vi "Arm Motor Example.vi"() -> ()   [LabVIEW 2011]
panel:
  in  "Velocity":dbl(knob)=1.0440740470075023 scale=-10.0..10.0
  out "Motor Power":dbl(slide) scale=-1.0..1.0
  out "Waveform Chart":dbl(graph)
  in  "initialize":bool
  out "Position":dbl format="%0.2f"
  in  "Right/Up/CW Limit":dbl=10.0
  in  "Left/Dn/CCW Limit":dbl=-10.0
  in  "Joystick Input":dbl(slide)=0.005128205128205127 scale=-1.0..1.0
  out "Motor":dbl
  out "Read Right Limit":dbl=30.0
  out "Read Left Limit":dbl=-185.0
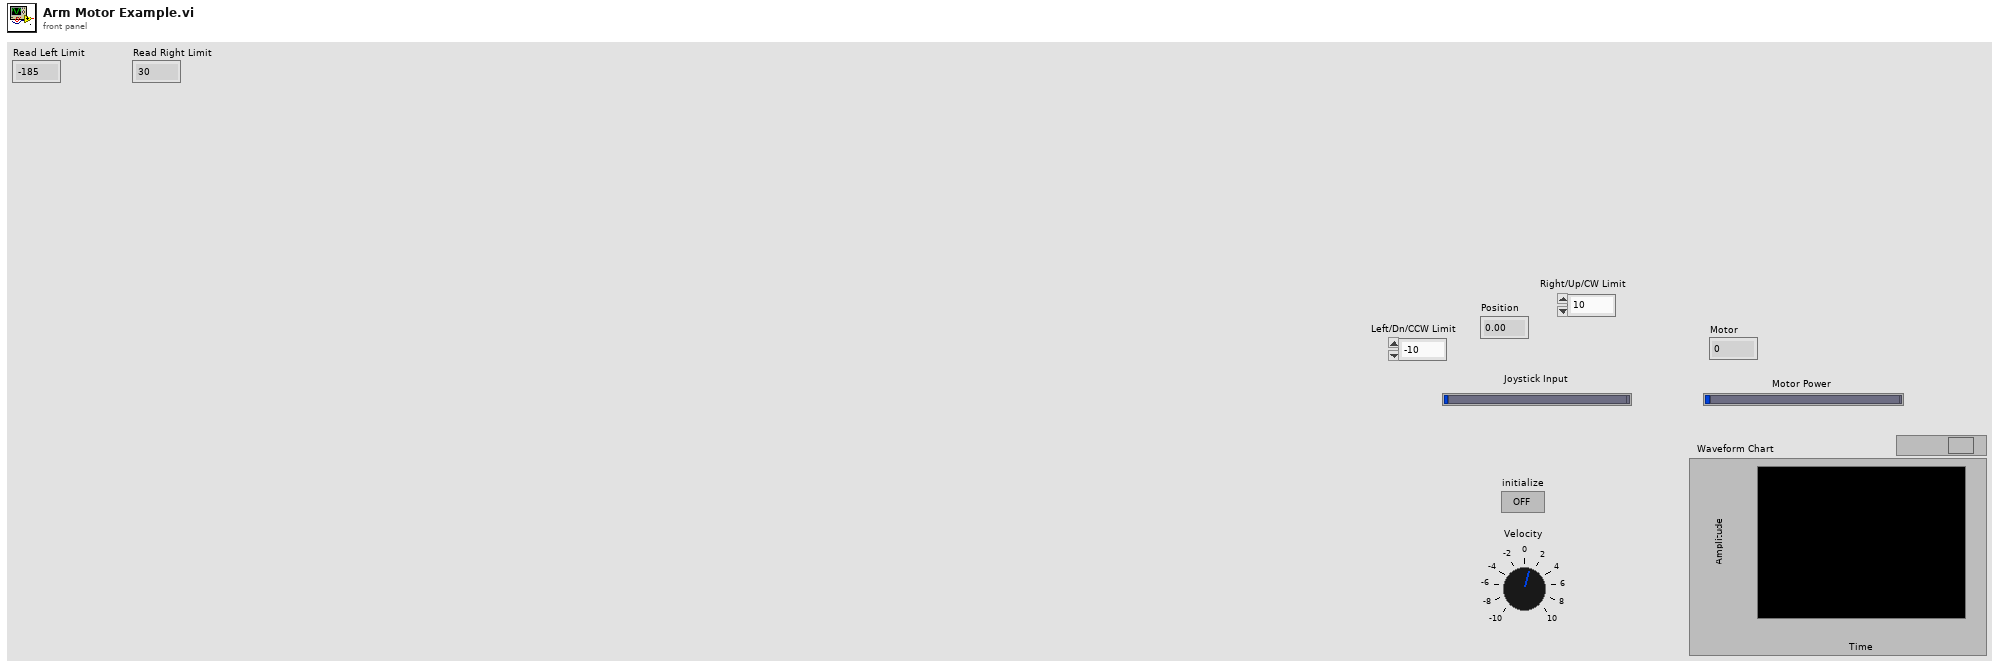
[diagram p1: front panel]
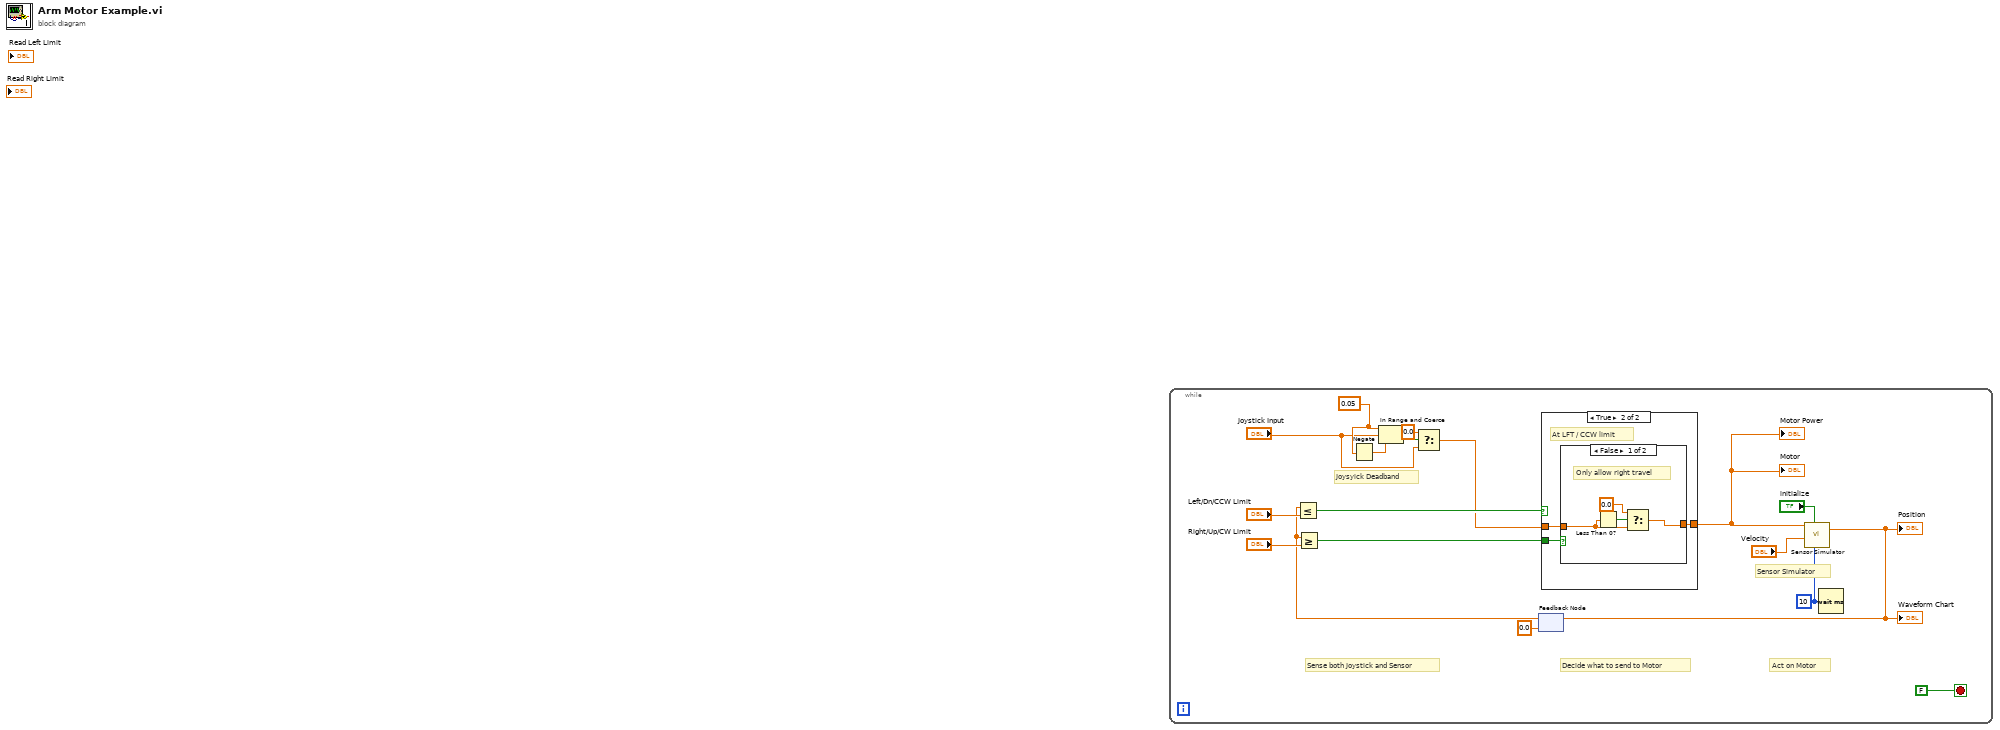
[diagram p0: block diagram]
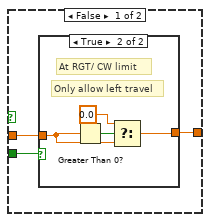
[diagram p2: hidden frame]
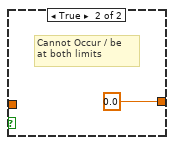
[diagram p4: hidden frame]
diagram:
  n1 = while {
    stop <- FALSE stop-if-true
    w7 = 0.05 ("upper limit")
    w2 = u32 10 ("milliseconds to wait")
    # "Act on Motor"
    # "Decide what to send to Motor"
    # "Sense both Joystick and Sensor"
    # "Sensor Simulator"
    # "Joysyick Deadband"
    n2 = Negate(x=w7) -> (-x=w8:dbl)
    n3 = In Range and Coerce(upper limit=w7, x="Joystick Input", lower limit=w8) -> (In Range?=w6:bool)  [unwired: 1 out]
    n4 = Select(t=0.0, s=w6, f="Joystick Input") -> (s? t:f=w5:dbl)
    n5 = feedback #1(0.0 ("Position")) -> (w13:dbl)
    n6 = Less Or Equal?(x=w13, y="Left/Dn/CCW Limit") -> (x <= y?=w18:bool)
    n7 = Greater Or Equal?(x=w13, y="Right/Up/CW Limit") -> (x >= y?=w17:bool)
    n8 = case shown="True" w18 {
      tunnel: [w21 w29] -> w12
      tunnel: w17 -> [w19 w28]
      tunnel: w5 -> [w20 w27]
      frame False {
        n9 = case shown="True" w19 {
          tunnel: [w22 w24] -> w21
          tunnel: w20 -> [w22 w23]
          frame False {
            # "At neither limit"
          }
          frame True {
            # "Only allow left travel"
            # "At RGT/ CW limit"
            n10 = Greater Than 0?(x=w23) -> (x > 0?=w26:bool)
            n11 = Select(t=0.0, s=w26, f=w23) -> (s? t:f=w24:dbl)
          }
        }
      }
      frame True {
        # "At LFT / CCW limit"
        n12 = case shown="False" w28 {
          tunnel: [w31 0.0 ("Turret Yaw Control")] -> w29
          tunnel: w27 -> [w30 _]
          frame False {
            # "Only allow right travel"
            n13 = Less Than 0?(x=w30) -> (x < 0?=w33:bool)
            n14 = Select(t=0.0, s=w33, f=w30) -> (s? t:f=w31:dbl)
          }
          frame True {
            # "Cannot Occur / be \nat both limits"
          }
        }
      }
    }
    "Motor" <- w12
    "Motor Power" <- w12
    n15 = call "Sensor Simulator.vi"("Loop Rate (ms)"=w2, "initialize"="initialize", "Velocity"="Velocity", "Input"=w12) -> ("Position"=w9:dbl)  [unwired: 3 in]
    "Position" <- w9
    "Waveform Chart" <- w9
    n16 = feedback-in #1(w9) -> ()
    n17 = Wait (ms)(milliseconds to wait=w2) -> ()  [unwired: 1 out]
  }
